vi "GetEnumFeatureEntrys.vi"(7 "handle":i64, 9 "EntryNum":u32, 10 "pFeatureName":string, 11 "error in (no error)":errorcluster) -> (1 "return type":i32, 2 "pLbEnumEntryList out":string, 3 "error out":errorcluster)   [LabVIEW 2016]
uses:
  MVSDKmd.dll
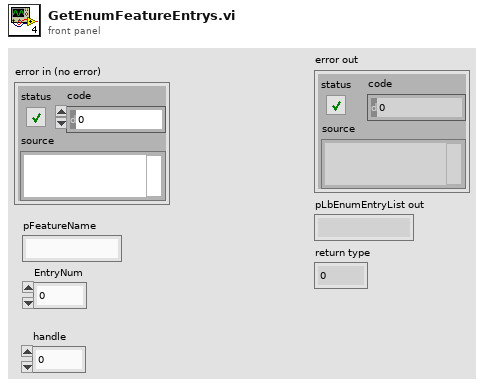
[diagram p1: front panel]
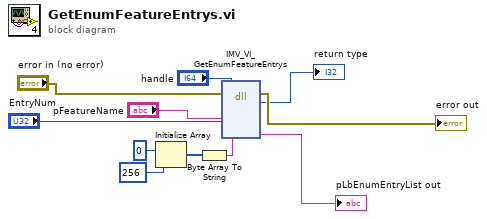
[diagram p0: block diagram]
diagram:
  n1 = Initialize Array(u8 0 ("element"), 256 ("dimension size")) -> (w2:u8[])
  n2 = Byte Array To String(unsigned byte array=w2) -> (string=w1:string)
  n3 = dll-call lib="MVSDKmd.dll" fn="IMV_VI_GetEnumFeatureEntrys"(error in="error in (no error)", "handle"="handle", "pFeatureName"="pFeatureName", "EntryNum"="EntryNum", "pLbEnumEntryList"=w1) -> (error out=→"error out":errorcluster, "return type"=→"return type":i32, "pLbEnumEntryList"=→"pLbEnumEntryList out":string)  [unwired: 5 in, 1 out]
